vi "Maglev_Main_VI_v1.vi"() -> ()   [LabVIEW 2017]
uses:
  <vilib>/eio/EIONode/EIONode.xnode
  <vilib>/rvi/eio/common/nirviEmuTemplateMethod_errors.vi
  <vilib>/rvi/DataTransferAndStorage/Container/XNode/niFpgaContainer.xnode
  <vilib>/rvi/FIFO/Fifo_Resource/nirvififoEmulationWrite.vi
  <vilib>/rvi/FIFO/Fifo_Resource/nirvififoEmulationRead.vi
  Components/FPGA Functions/FPGA functions.lvlib
panel:
  in  "AO loop time (Ticks)":u16=322
  in  "Control loop time (Ticks)":u8=8 caption="Control time (Ticks)"
  in  "AI loop time":u8=240 caption="AI loop time (Ticks)"
  out "AO loop time [ticks]":u16
  out "Controller loop time":u8
  out "AI proc. time [ticks]":u8
  out "Sample Freq. \ntoo high?":bool
  out "AI Loop time [ticks]":u8
  out "FPGA AI FIFO\nOverflow?":bool
  out "Hall3 [V]":fxp<+,25,3> format="%#.8g"
  out "Hall2 [V]":fxp<+,25,3> format="%#.8g"
  out "Hall1 [V]":fxp<+,25,3> format="%#.8g"
  in  "AO Coil3":u16
  in  "AO Coil2":u16
  in  "AO Coil1":u16
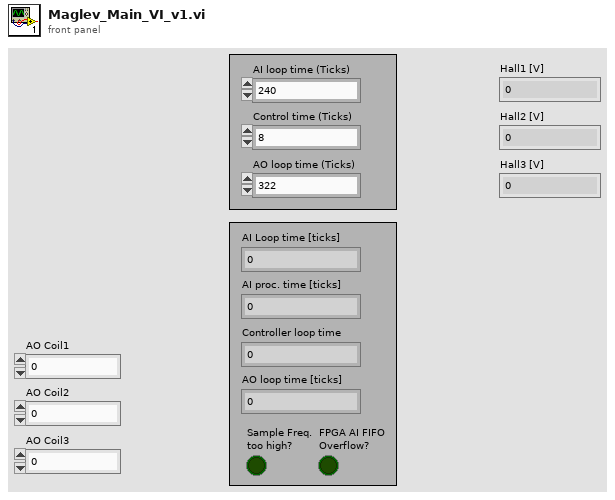
[diagram p1: front panel]
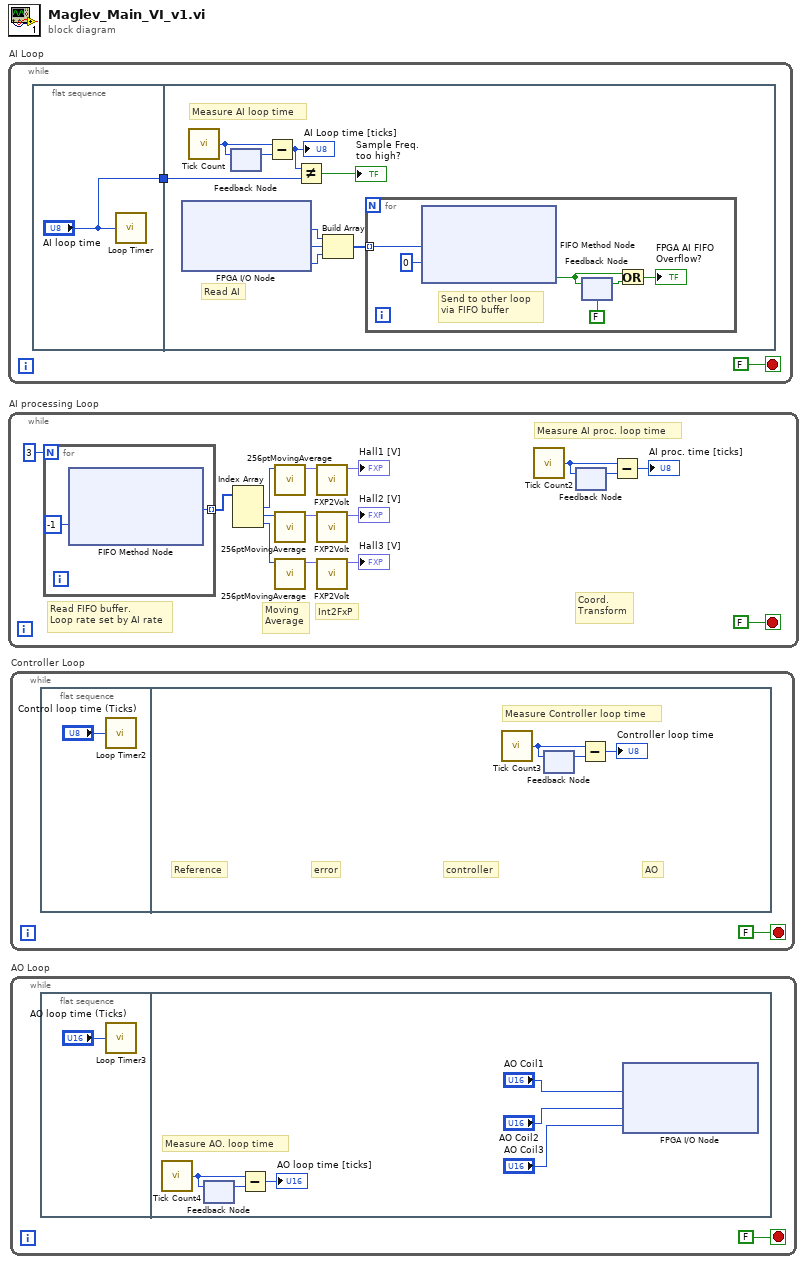
[diagram p0: block diagram]
diagram:
  n1 = while "AI Loop" {
    stop <- FALSE stop-if-true
    n2 = flat-sequence {
      tunnel: ["AI loop time"] -> w1
      tunnel: w1 -> [w4]
      frame #0 {
        n3 = call "Loop Timer"("Count(Ticks)"="AI loop time") -> ()  [unwired: 1 out]
      }
      frame #1 {
        # "Read AI"
        # "Measure AI loop time"
        n4 = xnode "FPGA I/O Node"() -> ("ConnectorA/AI0"=w12:u16, "ConnectorB/AI0"=w10:u16, "ConnectorB/AI1"=w11:u16)  [unwired: 3 in, 3 out]
        n5 = call "Tick Count"() -> ("Tick Count(Ticks)"=w8:u8)
        n6 = feedback #1() -> (w7:u8)  [unwired: 1 in]
        n7 = feedback-in #1(w8) -> ()
        n8 = Subtract(x=w8, y=w7) -> (x-y=w6:u8)
        "AI Loop time [ticks]" <- w6
        n9 = Not Equal?(x=w6, y=w4) -> (x != y?=→"Sample Freq. \ntoo high?":bool)
        n10 = Build Array(w12, w10, w11) -> (w9:u16[])
        n11 = for {
          tunnel: w9 -> [w18] mode=indexing
          # "Send to other loop \nvia FIFO buffer"
          n12 = xnode ("FIFO Method Node")("Element"=w18, "Timeout"=0) -> ("Timed Out?"=w14:bool)  [unwired: 1 in, 1 out]
          n13 = feedback #2(FALSE ("Timed Out?")) -> (w15:bool)
          n14 = feedback-in #2(w14) -> ()
          n15 = Or(x=w14, y=w15) -> (x .or. y?=→"FPGA AI FIFO\nOverflow?":bool)
        }
      }
    }
  }
  n16 = while "AI processing Loop" {
    stop <- FALSE stop-if-true
    # "Measure AI proc. loop time"
    # "Read FIFO buffer.\nLoop rate set by AI rate"
    # "Coord.\nTransform"
    # "Int2FxP"
    # "Moving\nAverage"
    n17 = for {
      N: 3 -> [_]
      tunnel: [w34] -> w31 mode=indexing
      n18 = xnode ("FIFO Method Node")("Timeout"=-1) -> ("Element"=w34:u16)  [unwired: 1 in, 2 out]
    }
    n19 = Index Array(array=w31) -> (element #1=w30:u16, element #2=w29:u16, element #3=w28:u16)  [unwired: 3 in]
    n20 = call "256ptMovingAverage.vi"("Raw input"=w30) -> ("Avg. output"=w27:fxp<+,22,12>)  [unwired: 10 in]
    n21 = call "256ptMovingAverage.vi"("Raw input"=w29) -> ("Avg. output"=w26:fxp<+,22,12>)  [unwired: 10 in]
    n22 = call "256ptMovingAverage.vi"("Raw input"=w28) -> ("Avg. output"=w25:fxp<+,22,12>)  [unwired: 10 in]
    n23 = call "FXP2Volt.vi"("Input (Int)"=w27) -> ("Output (FXP)"=→"Hall1 [V]":fxp<+,25,3>)  [unwired: 10 in]
    n24 = call "FXP2Volt.vi"("Input (Int)"=w26) -> ("Output (FXP)"=→"Hall2 [V]":fxp<+,25,3>)  [unwired: 10 in]
    n25 = call "FXP2Volt.vi"("Input (Int)"=w25) -> ("Output (FXP)"=→"Hall3 [V]":fxp<+,25,3>)  [unwired: 10 in]
    n26 = call "Tick Count2"() -> ("Tick Count(Ticks)"=w21:u8)
    n27 = feedback #3() -> (w20:u8)  [unwired: 1 in]
    n28 = feedback-in #3(w21) -> ()
    n29 = Subtract(x=w21, y=w20) -> (x-y=→"AI proc. time [ticks]":u8)
  }
  n30 = while "Controller Loop" {
    stop <- FALSE stop-if-true
    n31 = flat-sequence {
      frame #0 {
        n32 = call "Loop Timer2"("Count(Ticks)"="Control loop time (Ticks)") -> ()  [unwired: 1 out]
      }
      frame #1 {
        # "Measure Controller loop time"
        # "AO"
        # "controller"
        # "error"
        # "Reference"
        n33 = call "Tick Count3"() -> ("Tick Count(Ticks)"=w40:u8)
        n34 = feedback #4() -> (w39:u8)  [unwired: 1 in]
        n35 = feedback-in #4(w40) -> ()
        n36 = Subtract(x=w40, y=w39) -> (x-y=→"Controller loop time":u8)
      }
    }
  }
  n37 = while "AO Loop" {
    stop <- FALSE stop-if-true
    n38 = flat-sequence {
      frame #0 {
        n39 = call "Loop Timer3"("Count(Ticks)"="AO loop time (Ticks)") -> ()  [unwired: 1 out]
      }
      frame #1 {
        # "Measure AO. loop time"
        n40 = call "Tick Count4"() -> ("Tick Count(Ticks)"=w45:u16)
        n41 = feedback #5() -> (w44:u16)  [unwired: 1 in]
        n42 = feedback-in #5(w45) -> ()
        n43 = Subtract(x=w45, y=w44) -> (x-y=→"AO loop time [ticks]":u16)
        n44 = xnode "FPGA I/O Node"("ConnectorA/AO0"="AO Coil1", "ConnectorB/AO0"="AO Coil2", "ConnectorB/AO1"="AO Coil3") -> ()  [unwired: 3 in, 3 out]
      }
    }
  }
